vi "ResetSolenoid.vi"(8 "error in (no error)":errorcluster, 11 "Solenoids in":refnum<class "Solenoids.lvclass">) -> (0 "error out":errorcluster, 3 "Solenoids out":refnum<class "Solenoids.lvclass">)   [LabVIEW 2019, in "Pneumatics control.lvlib" / "Solenoids.lvclass"]
doc: "This VI resets the solonoid."
uses:
  Solenoids.lvclass
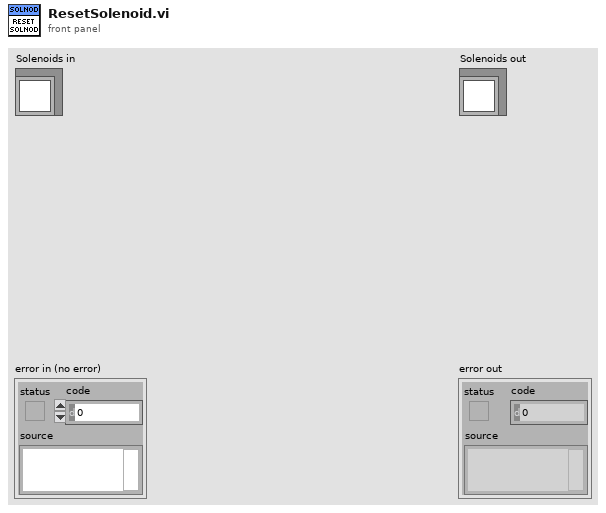
[diagram p1: front panel]
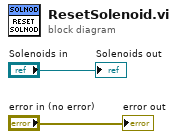
[diagram p0: block diagram]
diagram:
  "error out" <- "error in (no error)"
  "Solenoids out" <- "Solenoids in"
